vi "Format DC Pins to TestStand Array.vi"(8 "error in (no error)":errorcluster, 11 "QPA Measurement in":refnum<class "QPA Measurement.lvclass">) -> (0 "error out":errorcluster, 1 "PAE Pins":string, 2 "DC Pins":string, 3 "QPA Measurement out":refnum<class "QPA Measurement.lvclass">)   [LabVIEW 2016, in "QPA Measurement.lvlib" / "QPA Measurement.lvclass"]
uses:
  QPA Measurement.lvclass
  QPA Measurement.lvclass/QPA Measurement.ctl
  Protected Methods/Read DC Pins.vi
  Protected Methods/Read PAE Pins.vi
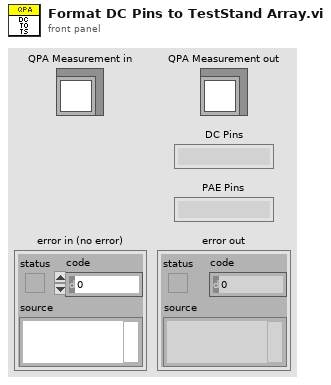
[diagram p1: front panel]
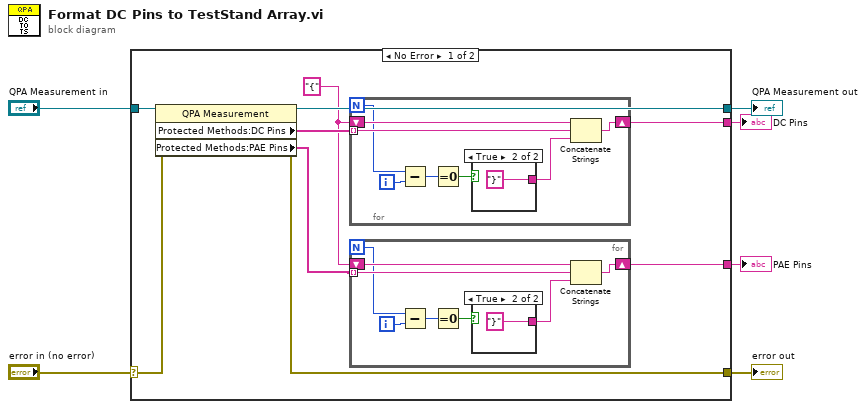
[diagram p0: block diagram]
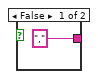
[diagram p2: hidden frame]
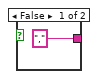
[diagram p3: hidden frame]
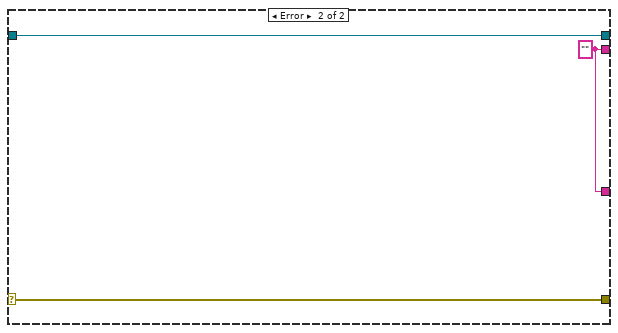
[diagram p4: hidden frame]
diagram:
  n1 = case shown="No Error" "error in (no error)" {
    selector: "error in (no error)" -> [w15 w38]
    tunnel: [w14 w38] -> w5
    tunnel: [w12 w37] -> w3
    tunnel: "QPA Measurement in" -> [w13 w37]
    tunnel: [w10 w36] -> w2
    tunnel: [w7 w36] -> w1
    frame No Error {
      w9 = "{"
      n2 = property class="QPA Measurement"(reference=w13, error in=w15) -> (reference out=w12:refnum<class "QPA Measurement.lvclass">, error out=w14:errorcluster, "Protected Methods:DC Pins"=w11:string[], "Protected Methods:PAE Pins"=w8:string[])
      n3 = for {
        N -> [w30]
        shift-right: [w31] -> w10
        shift-left: w9 -> [w32]
        tunnel: w11 -> [w33] mode=indexing
        i -> [w29]
        n4 = Subtract(x=w30, y=w29) -> (x-y=w28:i32)
        n5 = Equal To 0?(x=w28) -> (x = 0?=w27:bool)
        n6 = case shown="True" w27 {
          tunnel: ["," "}"] -> w26
          frame False {
          }
          frame True {
          }
        }
        n7 = Concatenate Strings(w32, w33, w26) -> (w31:string)
      }
      n8 = for {
        N -> [w20]
        shift-right: [w21] -> w7
        shift-left: w9 -> [w22]
        tunnel: w8 -> [w23] mode=indexing
        i -> [w19]
        n9 = Subtract(x=w20, y=w19) -> (x-y=w18:i32)
        n10 = Equal To 0?(x=w18) -> (x = 0?=w17:bool)
        n11 = case shown="True" w17 {
          tunnel: ["," "}"] -> w16
          frame False {
          }
          frame True {
          }
        }
        n12 = Concatenate Strings(w22, w23, w16) -> (w21:string)
      }
    }
    frame Error {
      w36 = ""
    }
  }
  "error out" <- w5
  "QPA Measurement out" <- w3
  "DC Pins" <- w2
  "PAE Pins" <- w1
